vi "Get Protocol_ex.vi"() -> ()   [LabVIEW 2019]
uses:
  <vilib>/NI VeriStand/Custom Device API/Custom Device Item Ref.ctl
  Addon/Support Libraries/Protocols.lvlibp/Protocol Parent/Protocol Parent.lvclass
  Scripting API/Scripting API.lvlib
  <vilib>/NI VeriStand/Custom Device API/Custom Device API.lvlib
panel:
  out "instrument addon refnum out":T1=18446744073709551615 format="%.0x"
  out "protocol":refnum<class "Protocol Parent.lvclass">
  out "error out":errorcluster
  in  "instrument addon refnum in":T1=18446744073709551615 format="%.0x"
  in  "error in (no error)":errorcluster
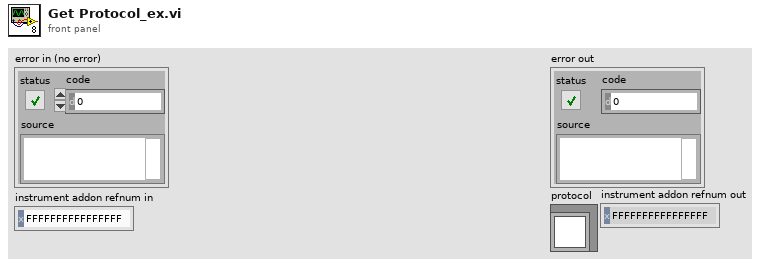
[diagram p1: front panel]
types:
  T1 = typedef "Custom Device API.lvlib/Custom Device Item Ref.ctl" = u64
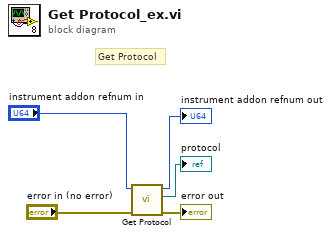
[diagram p0: block diagram]
diagram:
  # "Get Protocol"
  n1 = call "Get Protocol.vi"("error in (no error)"="error in (no error)", "instrument addon refnum in"="instrument addon refnum in") -> ("error out"=→"error out":errorcluster, "protocol"=→"protocol":refnum<class "Protocol Parent.lvclass">, "instrument addon refnum out"=→"instrument addon refnum out":T1)  [unwired: 7 in]
